vi "创建数据表.vi"(8 "error in (no error)":errorcluster) -> (0 "error out":errorcluster)   [LabVIEW 2016, in "数据查询.lvlib"]
uses:
  <vilib>/addons/database/Auxilliary.llb/DB Tools Column Info.ctl
  <vilib>/addons/database/Auxilliary.llb/DB Tools DataTypes.ctl
  <vilib>/addons/database/Connection.llb/DB Tools Open Connec (String).vi
  <userlib>/_LVST/sqlite_api/Core/Tables/SQLite_Drop Table.vi
  <userlib>/_LVST/sqlite_api/Core/Tables/SQLite_Create Table.vi
  <vilib>/addons/database/NI_Database_API.lvlib
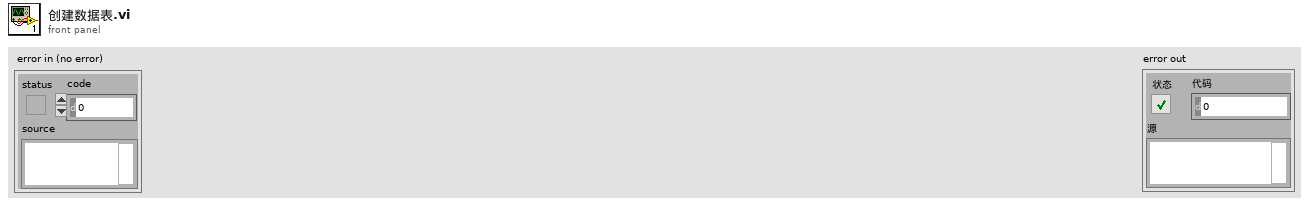
[diagram p1: front panel]
types:
  T1 = typedef "NI_Database_API.lvlib/DB Tools Column Info.ctl" = cluster{"column name":string, "data type":T2, "size":i32, "allow null?":bool}
  T2 = typedef "NI_Database_API.lvlib/DB Tools DataTypes.ctl" = enum16{"String", "Long (I32)", "Single (SGL)", "Double (DBL)", "Date/Time", "Binary"}
  T3 = typedef "NI_Database_API.lvlib/Conn ObjectReference.ctl" = refnum<k1>
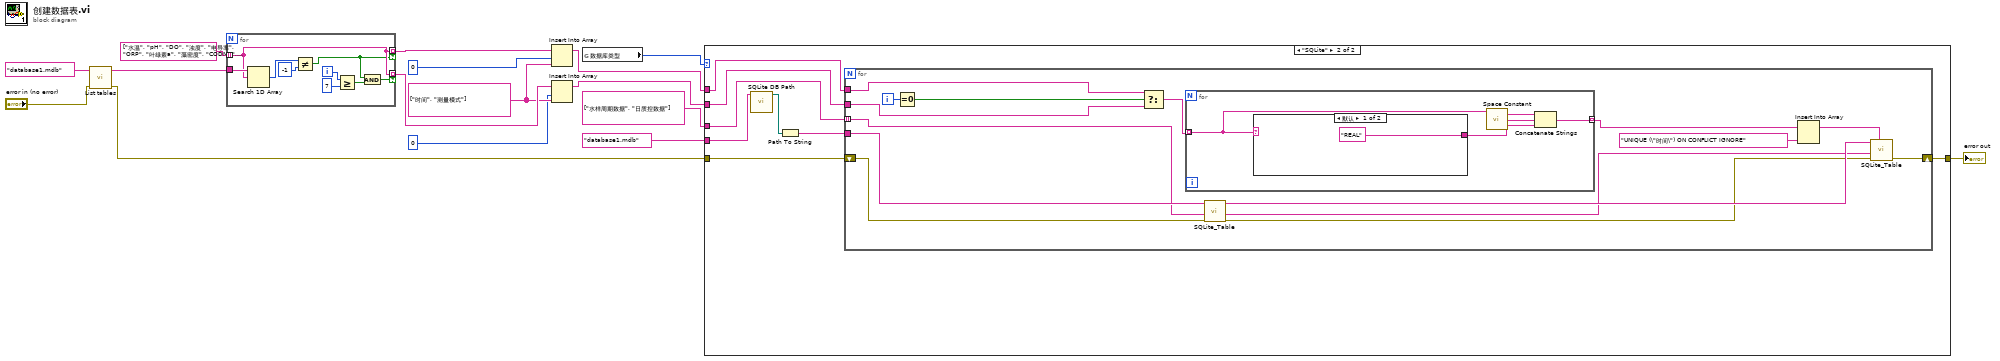
[diagram p0: block diagram]
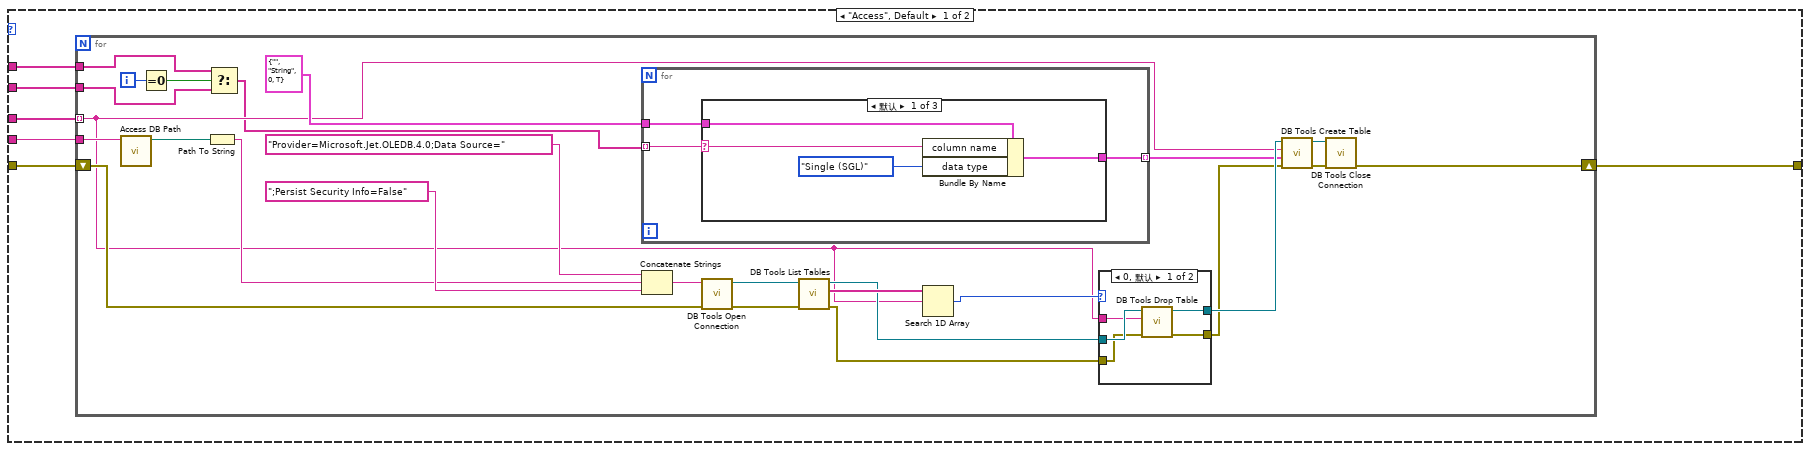
[diagram p2: hidden frame]
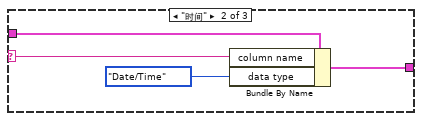
[diagram p3: hidden frame]
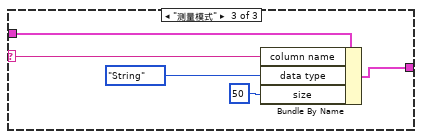
[diagram p4: hidden frame]
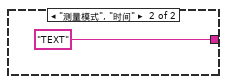
[diagram p6: hidden frame]
diagram:
  w11 = string[] ["时间", "测量模式"]
  n1 = call "List tables.vi"("error in (no error)"="error in (no error)", "database"="database1.mdb") -> ("error out"=w7:errorcluster, "tables"=w16:string[])  [unwired: 8 in]
  n2 = for {
    tunnel: string[] ["水温", "pH", "DO", "浊度", "电导率", "ORP", "叶绿素a", "藻密度", "CODMn", "CODcr", "COD", "磷酸盐", "氨氮", "总磷", "总氮", "亚硝氮", "硫化物", "硝氮", "硅酸盐"] -> [w22] mode=indexing
    tunnel: w16 -> [w25]
    tunnel: [w22] -> w15 mode=indexing if=w17
    tunnel: [w22] -> w12 mode=indexing if=w18
    i -> [w21]
    n3 = Search 1D Array(1D array=w25, element=w22) -> (index of element=w24:i32)  [unwired: 1 in]
    n4 = Not Equal?(x=w24, y=-1 ("x")) -> (x != y?=w17:bool)
    n5 = Greater Or Equal?(x=w21, y=7) -> (x >= y?=w19:bool)
    n6 = And(x=w17, y=w19) -> (x .and. y?=w18:bool)
  }
  n7 = Insert Into Array(array=w15, index=0 ("索引"), new element=w11) -> (w6:string[])
  n8 = Insert Into Array(array=w12, index=0 ("索引"), new element=w11) -> (w3:string[])
  n9 = global read "全局变量.vi" "数据库类型"() -> (w8:enum16{"Access", "SQLite"})
  n10 = case shown="\"SQLite\"" w8 {
    tunnel: w6 -> [w31 w84]
    tunnel: w7 -> [w30 w81]
    tunnel: [w29 w82] -> w1
    tunnel: "database1.mdb" ("database") -> [w28 w87]
    tunnel: string[] ["水样周期数据", "日质控数据"] -> [w27 w85]
    tunnel: w3 -> [w26 w83]
    frame "Access", Default {
      n11 = for {
        tunnel: w31 -> [w34]
        tunnel: w28 -> [w38]
        shift-right: [w39] -> w29
        shift-left: w30 -> [w40]
        tunnel: w27 -> [w37] mode=indexing
        tunnel: w26 -> [w33]
        i -> [w36]
        n12 = call "Access DB Path.vi"("database"=w38) -> ("appended path"=w42:path)  [unwired: 10 in]
        n13 = Equal To 0?(x=w36) -> (x = 0?=w35:bool)
        n14 = Path To String(path=w42) -> (string=w43:string)
        n15 = Select(t=w34, s=w35, f=w33) -> (s? t:f=w32:string[])
        n16 = for {
          tunnel: w32 -> [w60] mode=indexing
          tunnel: T1 {"column name"="", "data type"=enum."String", "size"=0, "allow null?"=TRUE} ("column information") -> [w59]
          tunnel: [w58] -> w46 mode=indexing
          n17 = case shown="默认" w60 {
            selector: w60 -> [w63 w67 w72]
            tunnel: w59 -> [w64 w68 w73]
            tunnel: [w62 w66 w71] -> w58
            frame Default {
              n18 = Bundle By Name(cluster=w64, "column name"=w63, "data type"=DB_Tools_DataTypes."Single (SGL)") -> (w62:T1)
            }
            frame "时间" {
              n19 = Bundle By Name(cluster=w68, "column name"=w67, "data type"=DB_Tools_DataTypes."Date/Time") -> (w66:T1)
            }
            frame "测量模式" {
              n20 = Bundle By Name(cluster=w73, "column name"=w72, "data type"=DB_Tools_DataTypes."String", "size"=50) -> (w71:T1)
            }
          }
        }
        n21 = Concatenate Strings("Provider=Microsoft.Jet.OLEDB.4.0;Data Source=" ("condition"), w43, ";Persist Security Info=False" ("condition")) -> (w41:string)
        n22 = call-poly <vilib>:"DB Tools Open Connection.vi"("error in (no error)"=w40, "connection information"=w41) -> ("error out"=w57:errorcluster, "connection reference"=w56:T3)  [unwired: 6 in]
        n23 = call <vilib>:"DB Tools List Tables.vi"("error in (no error)"=w57, "connection reference"=w56) -> ("error out"=w51:errorcluster, "tables"=w55:string[], "connection reference out"=w53:T3)  [unwired: 3 in]
        n24 = Search 1D Array(1D array=w55, element=w37) -> (index of element=w54:i32)  [unwired: 1 in]
        n25 = case shown="0, 默认" w54 {
          tunnel: w53 -> [w78 w80]
          tunnel: [w77 w80] -> w52
          tunnel: w51 -> [w76 w79]
          tunnel: [w75 w79] -> w50
          tunnel: w37 -> [w74 _]
          frame 0, Default {
            n26 = call <vilib>:"DB Tools Drop Table.vi"("error in (no error)"=w76, "table"=w74, "connection reference"=w78) -> ("error out"=w75:errorcluster, "connection reference out"=w77:T3)  [unwired: 5 in]
          }
          frame 1 {
          }
        }
        n27 = call <vilib>:"DB Tools Create Table.vi"("error in (no error)"=w50, "column information"=w46, "table"=w37, "connection reference"=w52) -> ("error out"=w48:errorcluster, "connection reference out"=w49:T3)  [unwired: 4 in]
        n28 = call <vilib>:"DB Tools Close Connection.vi"("error in (no error)"=w48, "connection reference"=w49) -> ("error out"=w39:errorcluster)  [unwired: 5 in]
      }
    }
    frame "SQLite" {
      n29 = call "SQLite DB Path.vi"("database"=w87) -> ("appended path"=w88:path)  [unwired: 10 in]
      n30 = Path To String(path=w88) -> (string=w86:string)
      n31 = for {
        tunnel: w86 -> [w101]
        tunnel: w85 -> [w100] mode=indexing
        tunnel: w84 -> [w96]
        tunnel: w83 -> [w95]
        shift-right: [w93] -> w82
        shift-left: w81 -> [w92]
        i -> [w98]
        n32 = Equal To 0?(x=w98) -> (x = 0?=w97:bool)
        n33 = Select(t=w96, s=w97, f=w95) -> (s? t:f=w94:string[])
        n34 = for {
          tunnel: w94 -> [w107] mode=indexing
          tunnel: [w104] -> w90 mode=indexing
          n35 = case shown="默认" w107 {
            tunnel: ["REAL" "TEXT"] -> w105
            frame Default {
            }
            frame "测量模式", "时间" {
            }
          }
          n36 = call <vilib>:"Space Constant.vi"() -> ("String"=w106:string)
          n37 = Concatenate Strings(w107, w106, w105) -> (w104:string)
        }
        n38 = call-poly <userlib>:"SQLite_Table.vi"("DB Path"=w101, "Table Name"=w100, "error in (no error)"=w92) -> ("DB Path Out"=w103:string, "Table Name Out"=w99:string, "error out"=w102:errorcluster)  [unwired: 5 in]
        n39 = Insert Into Array(array=w90, new element="UNIQUE (\"时间\") ON CONFLICT IGNORE" ("新元素/子数组")) -> (w89:string[])  [unwired: 1 in]
        n40 = call-poly <userlib>:"SQLite_Table.vi"("DB Path"=w103, "Table Name"=w99, "error in (no error)"=w102, "Columns"=w89) -> ("error out"=w93:errorcluster)  [unwired: 4 in, 2 out]
      }
    }
  }
  "error out" <- w1
